vi "Fetch Base Library Info.vi"(8 "Error in":errorcluster caption="Error in (no error)", 11 "Library in":refnum<vi>) -> (0 "Error out":errorcluster, 2 "Base Library Info":T1, 3 "Library out":refnum<vi>)   [LabVIEW 2023, in "VIDoc Parsing.lvlib"]
doc: "Fetches the base Library information"
uses:
  VIDoc Parsing.lvlib
  TypeDefs/Base Library Info Cluster.ctl
  <vilib>/picture/picture.llb/imagedata.ctl
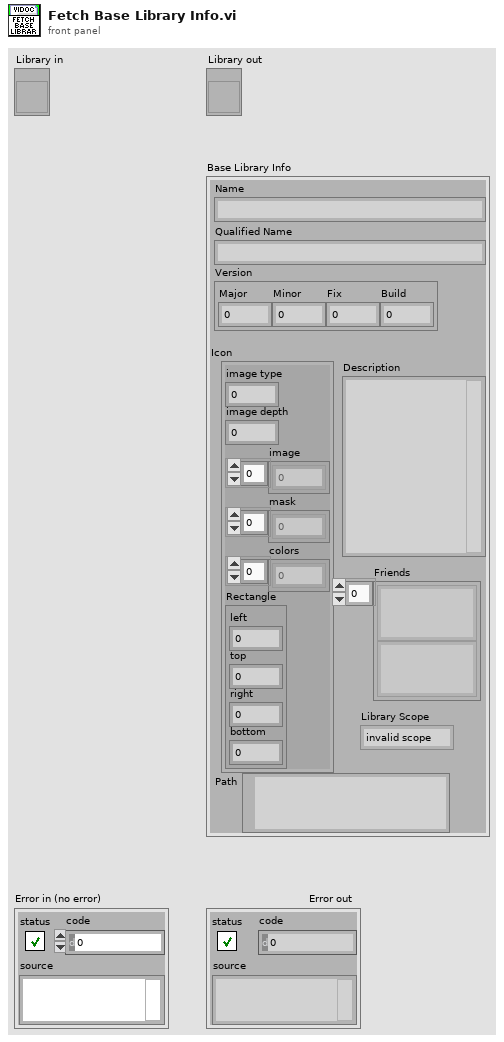
[diagram p1: front panel]
types:
  T1 = typedef "VIDoc Parsing.lvlib/Base Library Info Cluster.ctl" = cluster{"Name":string, "Icon":T2, "Version":cluster{"Major":u16, "Minor":u16, "Fix":u16, "Build":u16}, "Description":string, "Path":path, "Friends":string[], "Library Scope":enum32{"invalid scope", "public", "private", "protected", "community"}, "Qualified Name":string}
  T2 = typedef "imagedata.ctl" = cluster{"image type":i32, "image depth":i32, "image":u8[], "mask":u8[], "colors":u32[], "Rectangle":cluster{"left":i16, "top":i16, "right":i16, "bottom":i16}}
  T3 = enum32{"invalid scope", "public", "private", "protected", "community"}
  T4 = cluster{"Major":u16, "Minor":u16, "Fix":u16, "Build":u16}
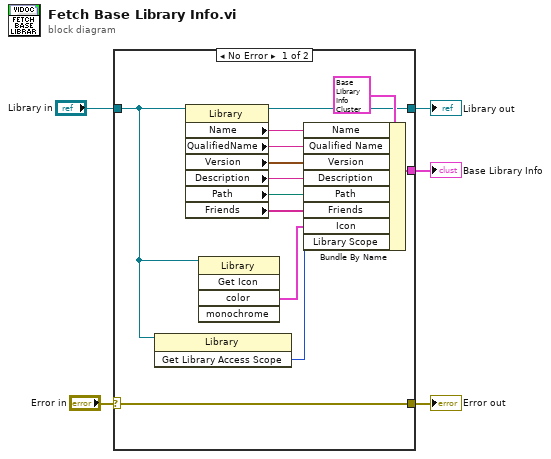
[diagram p0: block diagram]
diagram:
  n1 = case shown="No Error" "Error in" {
    selector: "Error in" -> [w10 w20]
    tunnel: "Library in" -> [w9 w19]
    tunnel: [w13 _] -> w4
    tunnel: [w12 w19] -> w3
    tunnel: [w10 w20] -> w2
    frame No Error {
      n2 = invoke class="Library" method="Get Library Access Scope"(reference=w9) -> ("Get Library Access Scope"=w8:T3)  [unwired: 2 in, 2 out]
      n3 = property class="Library"(reference=w9) -> (reference out=w12:refnum<vi>, "Name"=w16:string, "QualifiedName"=w6:string, "Version"=w17:T4, "Description"=w18:string, "Path"=w15:path, "Friends"=w11:string[])  [unwired: 1 in, 1 out]
      n4 = invoke class="Library" method="Get Icon"(reference=w9) -> ("color"=w7:T2)  [unwired: 4 in, 4 out]
      n5 = Bundle By Name(cluster=T1 {"Name"="", "Icon"={"image type"=0, "image depth"=0, "image"=[], "mask"=[], "colors"=[], "Rectangle"={"left"=0, "top"=0, "right"=0, "bottom"=0}}, "Version"={"Major"=0, "Minor"=0, "Fix"=0, "Build"=0}, "Description"="", "Path"=path "", "Friends"=[], "Library Scope"=enum."invalid scope", "Qualified Name"=""} ("Library Info"), "Name"=w16, "Qualified Name"=w6, "Version"=w17, "Description"=w18, "Path"=w15, "Friends"=w11, "Icon"=w7, "Library Scope"=w8) -> (w13:T1)
    }
    frame Error {
    }
  }
  "Base Library Info" <- w4
  "Library out" <- w3
  "Error out" <- w2
